vi "Dpc Set Def Port.vi"(8 "error in (no error)":errorcluster, 11 "prt":i32) -> (0 "error out":errorcluster, 3 "function return":i32)   [LabVIEW 2011, in "LVH-Adept.lvlib" / "DPCUTIL.lvlib"]
doc: "DPCAPI BOOL DpcSetDefPort(INT32 prt);"
uses:
  DPCUTIL.lvlib
  Resources/dpcutil.dll
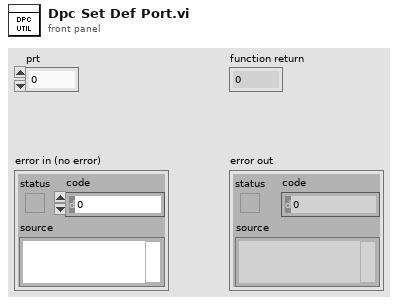
[diagram p1: front panel]
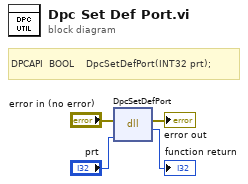
[diagram p0: block diagram]
diagram:
  # "DPCAPI  BOOL    DpcSetDefPort(INT32 prt);"
  n1 = dll-call lib="C:/github/labviewhacker/LVH-Adept/LabVIEW/vi.lib/LabVIEW Hacker/Adept/Private/Resources/dpcutil.*" fn="DpcSetDefPort"(error in="error in (no error)", "prt"="prt") -> (error out=→"error out":errorcluster, →"function return":i32)  [unwired: 3 in, 1 out]
